vi "Get Bits Per Digit from Base.vi"(11 "base":u8(ring)=10 items=["Binary (2)"=2, "Octal (8)"=8, "Decimal (10)"=10, "Hexadecimal (16)"=16]) -> (2 "bits per digit":i32, 3 "base out":i32)   [LabVIEW 2027, in "Encoding and Decoding.lvlib"]
doc: "Given the input base, returns the bits required for each digit of a value.\nb: 1\no: 3\nd: 4\nx: 4"
uses:
  Encoding and Decoding.lvlib
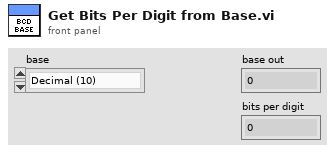
[diagram p1: front panel]
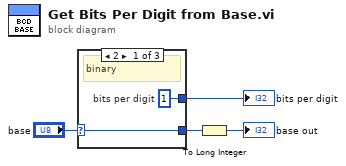
[diagram p0: block diagram]
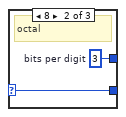
[diagram p2: hidden frame]
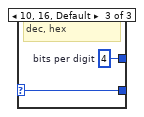
[diagram p3: hidden frame]
diagram:
  n1 = case shown="2" "base" {
    selector: "base" -> [w6 w8 w10]
    tunnel: [w6 w8 w10] -> w3
    tunnel: [w5 w7 w9] -> w2
    frame 2 {
      w5 = 1  # bits per digit
      # "binary"
    }
    frame 8 {
      w7 = 3  # bits per digit
      # "octal"
    }
    frame 10, 16, Default {
      w9 = 4  # bits per digit
      # "dec, hex"
    }
  }
  "bits per digit" <- w2
  n2 = To Long Integer(number=w3) -> (32bit integer=→"base out":i32)
